vi "DBmaker.vi"(9 "DBname":string) -> (1 "IDs No":dbl, 3 "DBarray":dbl[][](array[numeric]))   [LabVIEW 2021]
panel:
  out "error out":errorcluster
  out "size(s)":i32[](array[numeric])
  out "concatenated string 2":string
  out "concatenated string":string
  in  "return value 2":dbl[][](array[numeric])
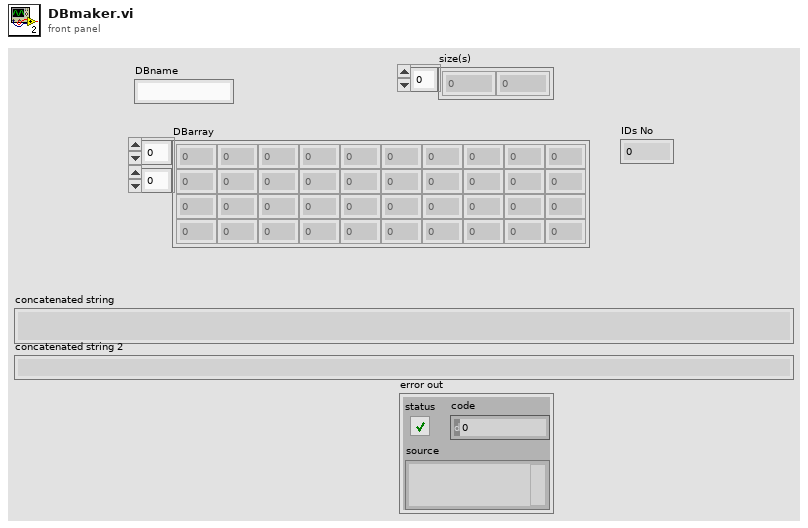
[diagram p1: front panel]
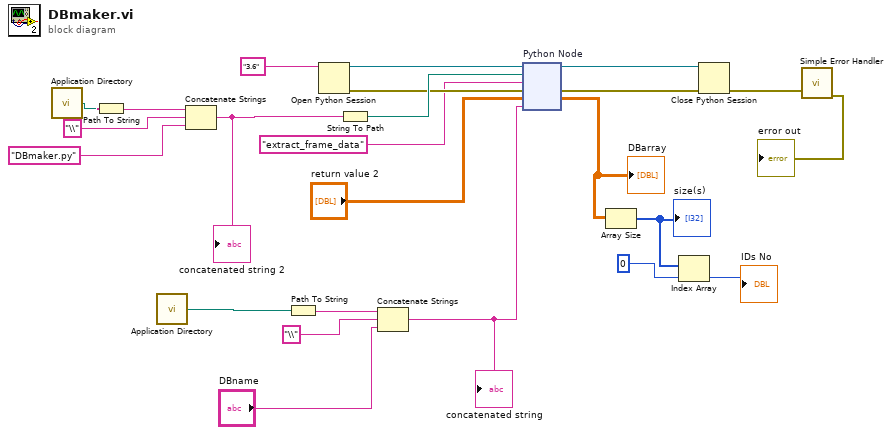
[diagram p0: block diagram]
diagram:
  n1 = call <vilib>:"Application Directory.vi"() -> ("Application Directory"=w9:path)
  n2 = Path To String(path=w9) -> (string=w11:string)
  n3 = call <vilib>:"Application Directory.vi"() -> ("Application Directory"=w16:path)
  n4 = Concatenate Strings(w11, "\\" ("string"), "DBmaker.py" ("string")) -> (w7:string)
  "concatenated string 2" <- w7
  n5 = Path To String(path=w16) -> (string=w15:string)
  n6 = Open Python Session(python version="3.6" ("Python version")) -> (session out=w23:refnum<k35>, error out=w20:errorcluster)  [unwired: 2 in]
  n7 = String To Path(string=w7) -> (path=w24:path)
  n8 = Concatenate Strings(w15, "\\" ("string"), "DBname") -> (w14:string)
  "concatenated string" <- w14
  n9 = node "Python Node"(w23, w24, "extract_frame_data" ("function name"), w20, "return value 2", w14) -> (w22:refnum<k35>, w21:errorcluster, w6:dbl[][])  [unwired: 1 in, 2 out]
  "DBarray" <- w6
  n10 = Array Size(array=w6) -> (size(s)=w3:i32[])
  "size(s)" <- w3
  n11 = Index Array(array=w3, index=0 ("index (row)")) -> (element=→"IDs No":i32)
  n12 = Close Python Session(session in=w22, error in=w21) -> (11:w2:errorcluster)
  n13 = call <vilib>:"Simple Error Handler.vi"("error in (no error)"=w2) -> ("error out"=→"error out":errorcluster)  [unwired: 4 in, 4 out]
